vi "诊断标定3.vi"(8 "CAN端口":u16(ring), 9 "设备索引号":u16(ring), 10 "CAN卡类型":u32(ring)=21) -> ()   [LabVIEW 2013] (continued)
            n2342 = global write "EV05全局变量1.vi" "流控帧 2"(TRUE ("流控帧 2")) -> ()
            n2343 = local write "写?"(FALSE ("写?")) -> ()
            n2344 = local write "消除"(TRUE ("消除")) -> ()
          }
          frame #2 {
            n2345 = flat-sequence {
              tunnel: [w2891] -> w2890
              tunnel: w2890 -> [w2898]
              frame #0 {
                n2346 = while {
                  tunnel: [w2892] -> w2891
                  i -> [w2896]
                  stop <- w2893 stop-if-true
                  n2347 = local read "继电器超时处理"() -> (w2892:bool)
                  n2348 = Greater Or Equal?(x=w2896, y=20) -> (x >= y?=w2894:bool)
                  n2349 = Wait Until Next ms Multiple(millisecond multiple=u32 100 ("毫秒倍数")) -> ()  [unwired: 1 out]
                  n2350 = Or(x=w2892, y=w2894) -> (x .or. y?=w2893:bool)
                }
              }
              frame #1 {
                n2351 = case shown="假" w2898 {
                  frame False {
                    n2352 = local read "负级继电器"() -> (w2899:bool)
                    n2353 = Not(x=w2899) -> (.not. x?=w2900:bool)
                    n2354 = local write "负级继电器"(w2900) -> ()
                    n2355 = One Button Dialog(message="继电器处理超时" ("消息"), button name ("OK")="是" ("按钮名称（“确定”）")) -> ()  [unwired: 1 out]
                  }
                  frame True {
                  }
                }
              }
            }
          }
        }
      }
      event "预充电继电器": Value Change {
        n2356 = event-data() -> ("NewVal"=w2903:bool)  [unwired: 6 out]
        n2357 = stacked-sequence {
          tunnel: w2903 -> [_ w2916 _]
          frame #0 {
            w2907 = FALSE ("继电器超时处理")
            n2358 = local write "继电器超时处理"(w2907) -> ()
            n2359 = local write "正级继电器 3"(w2907) -> ()
            n2360 = global write "EV05全局变量1.vi" "流控帧"(FALSE ("流控帧")) -> ()
            n2361 = local write "主从选择"(enum32{"主板", "从板"}."主板" ("主从选择")) -> ()
          }
          frame #1 {
            n2362 = case shown="假" w2916 {
              selector: w2916 -> [w2930 w2950]
              tunnel: [w2929 w2949] -> w2915
              tunnel: [w2918 w2938] -> w2910
              frame False {
                w2926 = 256.0 ("y")
                w2918 = u32 1 ("命令序号")
                w2929 = u8 192 ("命令")
                n2363 = local read "动作保持时间"() -> (w2927:dbl)
                n2364 = Quotient & Remainder(x=w2927, y=w2926) -> (x-y*floor(x/y)=w2919:dbl, floor(x/y)=w2923:dbl)
                n2365 = Quotient & Remainder(x=w2923, y=w2926) -> (x-y*floor(x/y)=w2920:dbl, floor(x/y)=w2924:dbl)
                n2366 = Quotient & Remainder(x=w2924, y=w2926) -> (x-y*floor(x/y)=w2921:dbl, floor(x/y)=w2925:dbl)
                n2367 = Quotient & Remainder(x=w2925, y=w2926) -> (x-y*floor(x/y)=w2922:dbl)  [unwired: 1 out]
                n2368 = Boolean To (0,1)(Boolean=w2930) -> (0, 1=w2928:i16)
                n2369 = local read "设备索引号"() -> (w2935:u16)
                n2370 = local read "CAN卡类型"() -> (w2936:u32)
                n2371 = local read "CAN端口"() -> (w2934:u16)
                n2372 = Build Array(i16 3 ("元素"), w2928, w2922, w2921, w2920, w2919, 0.0 ("元素")) -> (w2932:dbl[])
                n2373 = call "多帧发送机制(EV05).vi"("can卡类型"=w2936, "设备索引号"=w2935, "CAN端口"=w2934, "命令"=w2929, "板号"=u8 0, "命令序号"=w2918, "输入数据"=w2932) -> ()  [unwired: 1 in, 12 out]
              }
              frame True {
                w2946 = 256.0 ("y")
                w2938 = u32 1 ("命令序号")
                w2949 = u8 192 ("命令")
                n2374 = local read "动作保持时间"() -> (w2947:dbl)
                n2375 = Quotient & Remainder(x=w2947, y=w2946) -> (x-y*floor(x/y)=w2939:dbl, floor(x/y)=w2943:dbl)
                n2376 = Quotient & Remainder(x=w2943, y=w2946) -> (x-y*floor(x/y)=w2940:dbl, floor(x/y)=w2944:dbl)
                n2377 = Quotient & Remainder(x=w2944, y=w2946) -> (x-y*floor(x/y)=w2941:dbl, floor(x/y)=w2945:dbl)
                n2378 = Quotient & Remainder(x=w2945, y=w2946) -> (x-y*floor(x/y)=w2942:dbl)  [unwired: 1 out]
                n2379 = Boolean To (0,1)(Boolean=w2950) -> (0, 1=w2948:i16)
                n2380 = local read "设备索引号"() -> (w2955:u16)
                n2381 = local read "CAN卡类型"() -> (w2956:u32)
                n2382 = local read "CAN端口"() -> (w2954:u16)
                n2383 = Build Array(i16 3 ("元素"), w2948, w2942, w2941, w2940, w2939, 0.0 ("元素")) -> (w2952:dbl[])
                n2384 = call "多帧发送机制(EV05).vi"("can卡类型"=w2956, "设备索引号"=w2955, "CAN端口"=w2954, "命令"=w2949, "板号"=u8 0, "命令序号"=w2938, "输入数据"=w2952) -> ()  [unwired: 1 in, 12 out]
              }
            }
            n2385 = local write "命令序号"(w2910) -> ()
            n2386 = local write "清BUFF"(FALSE ("清BUFF")) -> ()
            n2387 = local write "控制1"(TRUE ("控制1")) -> ()
            n2388 = global write "EV05全局变量1.vi" "流控帧 2"(TRUE ("流控帧 2")) -> ()
            n2389 = local write "消除"(TRUE ("消除")) -> ()
            n2390 = local write "命令"(w2915) -> ()
            n2391 = local write "写?"(FALSE ("写?")) -> ()
          }
          frame #2 {
            n2392 = flat-sequence {
              tunnel: [w2958] -> w2957
              tunnel: w2957 -> [w2965]
              frame #0 {
                n2393 = while {
                  tunnel: [w2959] -> w2958
                  i -> [w2963]
                  stop <- w2960 stop-if-true
                  n2394 = local read "继电器超时处理"() -> (w2959:bool)
                  n2395 = Greater Or Equal?(x=w2963, y=20) -> (x >= y?=w2961:bool)
                  n2396 = Wait Until Next ms Multiple(millisecond multiple=u32 100 ("毫秒倍数")) -> ()  [unwired: 1 out]
                  n2397 = Or(x=w2959, y=w2961) -> (x .or. y?=w2960:bool)
                }
              }
              frame #1 {
                n2398 = case shown="假" w2965 {
                  frame False {
                    n2399 = local read "预充电继电器"() -> (w2966:bool)
                    n2400 = Not(x=w2966) -> (.not. x?=w2967:bool)
                    n2401 = local write "预充电继电器"(w2967) -> ()
                    n2402 = One Button Dialog(message="继电器处理超时" ("消息"), button name ("OK")="是" ("按钮名称（“确定”）")) -> ()  [unwired: 1 out]
                  }
                  frame True {
                  }
                }
              }
            }
          }
        }
      }
      event "加热继电器": Value Change {
        n2403 = event-data() -> ("NewVal"=w2970:bool)  [unwired: 6 out]
        n2404 = stacked-sequence {
          tunnel: w2970 -> [_ w2983 _]
          frame #0 {
            w2974 = FALSE ("继电器超时处理")
            n2405 = local write "继电器超时处理"(w2974) -> ()
            n2406 = local write "正级继电器 5"(w2974) -> ()
            n2407 = global write "EV05全局变量1.vi" "流控帧"(FALSE ("流控帧")) -> ()
            n2408 = local write "主从选择"(enum32{"主板", "从板"}."主板" ("主从选择")) -> ()
          }
          frame #1 {
            n2409 = case shown="假" w2983 {
              selector: w2983 -> [w2997 w3017]
              tunnel: [w2996 w3016] -> w2982
              tunnel: [w2985 w3005] -> w2977
              frame False {
                w2993 = 256.0 ("y")
                w2985 = u32 1 ("命令序号")
                w2996 = u8 192 ("命令")
                n2410 = local read "动作保持时间"() -> (w2994:dbl)
                n2411 = Quotient & Remainder(x=w2994, y=w2993) -> (x-y*floor(x/y)=w2986:dbl, floor(x/y)=w2990:dbl)
                n2412 = Quotient & Remainder(x=w2990, y=w2993) -> (x-y*floor(x/y)=w2987:dbl, floor(x/y)=w2991:dbl)
                n2413 = Quotient & Remainder(x=w2991, y=w2993) -> (x-y*floor(x/y)=w2988:dbl, floor(x/y)=w2992:dbl)
                n2414 = Quotient & Remainder(x=w2992, y=w2993) -> (x-y*floor(x/y)=w2989:dbl)  [unwired: 1 out]
                n2415 = Boolean To (0,1)(Boolean=w2997) -> (0, 1=w2995:i16)
                n2416 = local read "设备索引号"() -> (w3002:u16)
                n2417 = local read "CAN卡类型"() -> (w3003:u32)
                n2418 = local read "CAN端口"() -> (w3001:u16)
                n2419 = Build Array(i16 4 ("元素"), w2995, w2989, w2988, w2987, w2986, 0.0 ("元素")) -> (w2999:dbl[])
                n2420 = call "多帧发送机制(EV05).vi"("can卡类型"=w3003, "设备索引号"=w3002, "CAN端口"=w3001, "命令"=w2996, "板号"=u8 0, "命令序号"=w2985, "输入数据"=w2999) -> ()  [unwired: 1 in, 12 out]
              }
              frame True {
                w3013 = 256.0 ("y")
                w3005 = u32 1 ("命令序号")
                w3016 = u8 192 ("命令")
                n2421 = local read "动作保持时间"() -> (w3014:dbl)
                n2422 = Quotient & Remainder(x=w3014, y=w3013) -> (x-y*floor(x/y)=w3006:dbl, floor(x/y)=w3010:dbl)
                n2423 = Quotient & Remainder(x=w3010, y=w3013) -> (x-y*floor(x/y)=w3007:dbl, floor(x/y)=w3011:dbl)
                n2424 = Quotient & Remainder(x=w3011, y=w3013) -> (x-y*floor(x/y)=w3008:dbl, floor(x/y)=w3012:dbl)
                n2425 = Quotient & Remainder(x=w3012, y=w3013) -> (x-y*floor(x/y)=w3009:dbl)  [unwired: 1 out]
                n2426 = Boolean To (0,1)(Boolean=w3017) -> (0, 1=w3015:i16)
                n2427 = local read "设备索引号"() -> (w3022:u16)
                n2428 = local read "CAN卡类型"() -> (w3023:u32)
                n2429 = local read "CAN端口"() -> (w3021:u16)
                n2430 = Build Array(i16 4 ("元素"), w3015, w3009, w3008, w3007, w3006, 0.0 ("元素")) -> (w3019:dbl[])
                n2431 = call "多帧发送机制(EV05).vi"("can卡类型"=w3023, "设备索引号"=w3022, "CAN端口"=w3021, "命令"=w3016, "板号"=u8 0, "命令序号"=w3005, "输入数据"=w3019) -> ()  [unwired: 1 in, 12 out]
              }
            }
            n2432 = local write "命令序号"(w2977) -> ()
            n2433 = local write "清BUFF"(FALSE ("清BUFF")) -> ()
            n2434 = local write "命令"(w2982) -> ()
            n2435 = local write "控制1"(TRUE ("控制1")) -> ()
            n2436 = local write "写?"(FALSE ("写?")) -> ()
            n2437 = global write "EV05全局变量1.vi" "流控帧 2"(TRUE ("流控帧 2")) -> ()
            n2438 = local write "消除"(TRUE ("消除")) -> ()
          }
          frame #2 {
            n2439 = flat-sequence {
              tunnel: [w3025] -> w3024
              tunnel: w3024 -> [w3032]
              frame #0 {
                n2440 = while {
                  tunnel: [w3026] -> w3025
                  i -> [w3030]
                  stop <- w3027 stop-if-true
                  n2441 = local read "继电器超时处理"() -> (w3026:bool)
                  n2442 = Greater Or Equal?(x=w3030, y=20) -> (x >= y?=w3028:bool)
                  n2443 = Wait Until Next ms Multiple(millisecond multiple=u32 100 ("毫秒倍数")) -> ()  [unwired: 1 out]
                  n2444 = Or(x=w3026, y=w3028) -> (x .or. y?=w3027:bool)
                }
              }
              frame #1 {
                n2445 = case shown="假" w3032 {
                  frame False {
                    n2446 = local read "加热继电器"() -> (w3033:bool)
                    n2447 = Not(x=w3033) -> (.not. x?=w3034:bool)
                    n2448 = local write "加热继电器"(w3034) -> ()
                    n2449 = One Button Dialog(message="继电器处理超时" ("消息"), button name ("OK")="是" ("按钮名称（“确定”）")) -> ()  [unwired: 1 out]
                  }
                  frame True {
                  }
                }
              }
            }
          }
        }
      }
      event "充电继电器": Value Change {
        n2450 = event-data() -> ("NewVal"=w3037:bool)  [unwired: 6 out]
        n2451 = stacked-sequence {
          tunnel: w3037 -> [_ w3050 _]
          frame #0 {
            w3041 = FALSE ("继电器超时处理")
            n2452 = local write "主从选择"(enum32{"主板", "从板"}."主板" ("主从选择")) -> ()
            n2453 = global write "EV05全局变量1.vi" "流控帧"(FALSE ("流控帧")) -> ()
            n2454 = local write "继电器超时处理"(w3041) -> ()
            n2455 = local write "正级继电器 4"(w3041) -> ()
          }
          frame #1 {
            n2456 = case shown="假" w3050 {
              selector: w3050 -> [w3064 w3084]
              tunnel: [w3063 w3083] -> w3049
              tunnel: [w3052 w3072] -> w3044
              frame False {
                w3060 = 256.0 ("y")
                w3052 = u32 1 ("命令序号")
                w3063 = u8 192 ("命令")
                n2457 = local read "动作保持时间"() -> (w3061:dbl)
                n2458 = Quotient & Remainder(x=w3061, y=w3060) -> (x-y*floor(x/y)=w3053:dbl, floor(x/y)=w3057:dbl)
                n2459 = Quotient & Remainder(x=w3057, y=w3060) -> (x-y*floor(x/y)=w3054:dbl, floor(x/y)=w3058:dbl)
                n2460 = Quotient & Remainder(x=w3058, y=w3060) -> (x-y*floor(x/y)=w3055:dbl, floor(x/y)=w3059:dbl)
                n2461 = Quotient & Remainder(x=w3059, y=w3060) -> (x-y*floor(x/y)=w3056:dbl)  [unwired: 1 out]
                n2462 = Boolean To (0,1)(Boolean=w3064) -> (0, 1=w3062:i16)
                n2463 = local read "设备索引号"() -> (w3069:u16)
                n2464 = local read "CAN卡类型"() -> (w3070:u32)
                n2465 = local read "CAN端口"() -> (w3068:u16)
                n2466 = Build Array(i16 5 ("元素"), w3062, w3056, w3055, w3054, w3053, 0.0 ("元素")) -> (w3066:dbl[])
                n2467 = call "多帧发送机制(EV05).vi"("can卡类型"=w3070, "设备索引号"=w3069, "CAN端口"=w3068, "命令"=w3063, "板号"=u8 0, "命令序号"=w3052, "输入数据"=w3066) -> ()  [unwired: 1 in, 12 out]
              }
              frame True {
                w3080 = 256.0 ("y")
                w3072 = u32 1 ("命令序号")
                w3083 = u8 192 ("命令")
                n2468 = local read "动作保持时间"() -> (w3081:dbl)
                n2469 = Quotient & Remainder(x=w3081, y=w3080) -> (x-y*floor(x/y)=w3073:dbl, floor(x/y)=w3077:dbl)
                n2470 = Quotient & Remainder(x=w3077, y=w3080) -> (x-y*floor(x/y)=w3074:dbl, floor(x/y)=w3078:dbl)
                n2471 = Quotient & Remainder(x=w3078, y=w3080) -> (x-y*floor(x/y)=w3075:dbl, floor(x/y)=w3079:dbl)
                n2472 = Quotient & Remainder(x=w3079, y=w3080) -> (x-y*floor(x/y)=w3076:dbl)  [unwired: 1 out]
                n2473 = Boolean To (0,1)(Boolean=w3084) -> (0, 1=w3082:i16)
                n2474 = local read "设备索引号"() -> (w3089:u16)
                n2475 = local read "CAN卡类型"() -> (w3090:u32)
                n2476 = local read "CAN端口"() -> (w3088:u16)
                n2477 = Build Array(i16 5 ("元素"), w3082, w3076, w3075, w3074, w3073, 0.0 ("元素")) -> (w3086:dbl[])
                n2478 = call "多帧发送机制(EV05).vi"("can卡类型"=w3090, "设备索引号"=w3089, "CAN端口"=w3088, "命令"=w3083, "板号"=u8 0, "命令序号"=w3072, "输入数据"=w3086) -> ()  [unwired: 1 in, 12 out]
              }
            }
            n2479 = local write "命令序号"(w3044) -> ()
            n2480 = local write "命令"(w3049) -> ()
            n2481 = local write "清BUFF"(FALSE ("清BUFF")) -> ()
            n2482 = local write "控制1"(TRUE ("控制1")) -> ()
            n2483 = global write "EV05全局变量1.vi" "流控帧 2"(TRUE ("流控帧 2")) -> ()
            n2484 = local write "写?"(FALSE ("写?")) -> ()
            n2485 = local write "消除"(TRUE ("消除")) -> ()
          }
          frame #2 {
            n2486 = flat-sequence {
              tunnel: [w3092] -> w3091
              tunnel: w3091 -> [w3099]
              frame #0 {
                n2487 = while {
                  tunnel: [w3093] -> w3092
                  i -> [w3097]
                  stop <- w3094 stop-if-true
                  n2488 = local read "继电器超时处理"() -> (w3093:bool)
                  n2489 = Greater Or Equal?(x=w3097, y=20) -> (x >= y?=w3095:bool)
                  n2490 = Wait Until Next ms Multiple(millisecond multiple=u32 100 ("毫秒倍数")) -> ()  [unwired: 1 out]
                  n2491 = Or(x=w3093, y=w3095) -> (x .or. y?=w3094:bool)
                }
              }
              frame #1 {
                n2492 = case shown="假" w3099 {
                  frame False {
                    n2493 = local read "充电继电器"() -> (w3100:bool)
                    n2494 = Not(x=w3100) -> (.not. x?=w3101:bool)
                    n2495 = local write "充电继电器"(w3101) -> ()
                    n2496 = One Button Dialog(message="继电器处理超时" ("消息"), button name ("OK")="是" ("按钮名称（“确定”）")) -> ()  [unwired: 1 out]
                  }
                  frame True {
                  }
                }
              }
            }
          }
        }
      }
      event "风机继电器": Value Change {
        n2497 = event-data() -> ("NewVal"=w3104:bool)  [unwired: 6 out]
        n2498 = stacked-sequence {
          tunnel: w3104 -> [_ w3117 _]
          frame #0 {
            w3108 = FALSE ("继电器超时处理")
            n2499 = local write "继电器超时处理"(w3108) -> ()
            n2500 = local write "正级继电器 6"(w3108) -> ()
            n2501 = global write "EV05全局变量1.vi" "流控帧"(FALSE ("流控帧")) -> ()
            n2502 = local write "主从选择"(enum32{"主板", "从板"}."主板" ("主从选择")) -> ()
          }
          frame #1 {
            n2503 = case shown="真" w3117 {
              selector: w3117 -> [w3131 w3151]
              tunnel: [w3130 w3150] -> w3116
              tunnel: [w3119 w3139] -> w3111
              frame True {
                w3127 = 256.0 ("y")
                w3119 = u32 1 ("命令序号")
                w3130 = u8 192 ("命令")
                n2504 = local read "动作保持时间"() -> (w3128:dbl)
                n2505 = Quotient & Remainder(x=w3128, y=w3127) -> (x-y*floor(x/y)=w3120:dbl, floor(x/y)=w3124:dbl)
                n2506 = Quotient & Remainder(x=w3124, y=w3127) -> (x-y*floor(x/y)=w3121:dbl, floor(x/y)=w3125:dbl)
                n2507 = Quotient & Remainder(x=w3125, y=w3127) -> (x-y*floor(x/y)=w3122:dbl, floor(x/y)=w3126:dbl)
                n2508 = Boolean To (0,1)(Boolean=w3131) -> (0, 1=w3129:i16)
                n2509 = local read "设备索引号"() -> (w3136:u16)
                n2510 = local read "CAN卡类型"() -> (w3137:u32)
                n2511 = Quotient & Remainder(x=w3126, y=w3127) -> (x-y*floor(x/y)=w3123:dbl)  [unwired: 1 out]
                n2512 = local read "CAN端口"() -> (w3135:u16)
                n2513 = Build Array(i16 6 ("元素"), w3129, w3123, w3122, w3121, w3120, 0.0 ("元素")) -> (w3133:dbl[])
                n2514 = call "多帧发送机制(EV05).vi"("can卡类型"=w3137, "设备索引号"=w3136, "CAN端口"=w3135, "命令"=w3130, "板号"=u8 0, "命令序号"=w3119, "输入数据"=w3133) -> ()  [unwired: 1 in, 12 out]
              }
              frame False {
                w3147 = 256.0 ("y")
                w3139 = u32 1 ("命令序号")
                w3150 = u8 192 ("命令")
                n2515 = local read "动作保持时间"() -> (w3148:dbl)
                n2516 = Quotient & Remainder(x=w3148, y=w3147) -> (x-y*floor(x/y)=w3140:dbl, floor(x/y)=w3144:dbl)
                n2517 = Quotient & Remainder(x=w3144, y=w3147) -> (x-y*floor(x/y)=w3141:dbl, floor(x/y)=w3145:dbl)
                n2518 = Quotient & Remainder(x=w3145, y=w3147) -> (x-y*floor(x/y)=w3142:dbl, floor(x/y)=w3146:dbl)
                n2519 = Boolean To (0,1)(Boolean=w3151) -> (0, 1=w3149:i16)
                n2520 = local read "设备索引号"() -> (w3156:u16)
                n2521 = local read "CAN卡类型"() -> (w3157:u32)
                n2522 = Quotient & Remainder(x=w3146, y=w3147) -> (x-y*floor(x/y)=w3143:dbl)  [unwired: 1 out]
                n2523 = local read "CAN端口"() -> (w3155:u16)
                n2524 = Build Array(i16 6 ("元素"), w3149, w3143, w3142, w3141, w3140, 0.0 ("元素")) -> (w3153:dbl[])
                n2525 = call "多帧发送机制(EV05).vi"("can卡类型"=w3157, "设备索引号"=w3156, "CAN端口"=w3155, "命令"=w3150, "板号"=u8 0, "命令序号"=w3139, "输入数据"=w3153) -> ()  [unwired: 1 in, 12 out]
              }
            }
            n2526 = local write "命令序号"(w3111) -> ()
            n2527 = local write "命令"(w3116) -> ()
            n2528 = local write "清BUFF"(FALSE ("清BUFF")) -> ()
            n2529 = local write "控制1"(TRUE ("控制1")) -> ()
            n2530 = global write "EV05全局变量1.vi" "流控帧 2"(TRUE ("流控帧 2")) -> ()
            n2531 = local write "写?"(FALSE ("写?")) -> ()
            n2532 = local write "消除"(TRUE ("消除")) -> ()
          }
          frame #2 {
            n2533 = flat-sequence {
              tunnel: [w3159] -> w3158
              tunnel: w3158 -> [w3166]
              frame #0 {
                n2534 = while {
                  tunnel: [w3160] -> w3159
                  i -> [w3164]
                  stop <- w3161 stop-if-true
                  n2535 = local read "继电器超时处理"() -> (w3160:bool)
                  n2536 = Greater Or Equal?(x=w3164, y=20) -> (x >= y?=w3162:bool)
                  n2537 = Wait Until Next ms Multiple(millisecond multiple=u32 100 ("毫秒倍数")) -> ()  [unwired: 1 out]
                  n2538 = Or(x=w3160, y=w3162) -> (x .or. y?=w3161:bool)
                }
              }
              frame #1 {
                n2539 = case shown="假" w3166 {
                  frame False {
                    n2540 = local read "风机继电器"() -> (w3167:bool)
                    n2541 = Not(x=w3167) -> (.not. x?=w3168:bool)
                    n2542 = local write "风机继电器"(w3168) -> ()
                    n2543 = One Button Dialog(message="继电器处理超时" ("消息"), button name ("OK")="是" ("按钮名称（“确定”）")) -> ()  [unwired: 1 out]
                  }
                  frame True {
                  }
                }
              }
            }
          }
        }
      }
      event "加热继电器(从)": Value Change {
        n2544 = event-data() -> ("NewVal"=w3171:bool)  [unwired: 6 out]
        n2545 = stacked-sequence {
          tunnel: w3171 -> [_ w3185 _]
          frame #0 {
            w3175 = FALSE ("继电器超时处理")
            n2546 = local write "正级继电器 7"(w3175) -> ()
            n2547 = local write "继电器超时处理"(w3175) -> ()
            n2548 = global write "EV05全局变量1.vi" "流控帧"(FALSE ("流控帧")) -> ()
            n2549 = local write "主从选择"(enum32{"主板", "从板"}."从板" ("主从选择")) -> ()
          }
          frame #1 {
            n2550 = case shown="真" w3185 {
              selector: w3185 -> [w3200 w3220]
              tunnel: [w3199 w3219] -> w3184
              tunnel: [w3198 w3218] -> w3178
              tunnel: [w3187 w3207] -> w3179
              frame True {
                w3195 = 256.0 ("y")
                w3187 = u32 1 ("命令序号")
                w3199 = u8 192 ("命令")
                n2551 = local read "动作保持时间"() -> (w3196:dbl)
                n2552 = Quotient & Remainder(x=w3196, y=w3195) -> (x-y*floor(x/y)=w3188:dbl, floor(x/y)=w3192:dbl)
                n2553 = Quotient & Remainder(x=w3192, y=w3195) -> (x-y*floor(x/y)=w3189:dbl, floor(x/y)=w3193:dbl)
                n2554 = Quotient & Remainder(x=w3193, y=w3195) -> (x-y*floor(x/y)=w3190:dbl, floor(x/y)=w3194:dbl)
                n2555 = Quotient & Remainder(x=w3194, y=w3195) -> (x-y*floor(x/y)=w3191:dbl)  [unwired: 1 out]
                n2556 = Boolean To (0,1)(Boolean=w3200) -> (0, 1=w3197:i16)
                n2557 = local read "设备索引号"() -> (w3204:u16)
                n2558 = local read "CAN卡类型"() -> (w3205:u32)
                n2559 = local read "从板板号"() -> (w3198:u8)
                n2560 = local read "CAN端口"() -> (w3203:u16)
                n2561 = Build Array(i16 7 ("元素"), w3197, w3191, w3190, w3189, w3188, 0.0 ("元素")) -> (w3202:dbl[])
                n2562 = call "多帧发送机制(EV05).vi"("can卡类型"=w3205, "设备索引号"=w3204, "CAN端口"=w3203, "命令"=w3199, "板号"=w3198, "命令序号"=w3187, "输入数据"=w3202) -> ()  [unwired: 1 in, 12 out]
              }
              frame False {
                w3215 = 256.0 ("y")
                w3207 = u32 1 ("命令序号")
                w3219 = u8 192 ("命令")
                n2563 = local read "动作保持时间"() -> (w3216:dbl)
                n2564 = Quotient & Remainder(x=w3216, y=w3215) -> (x-y*floor(x/y)=w3208:dbl, floor(x/y)=w3212:dbl)
                n2565 = Quotient & Remainder(x=w3212, y=w3215) -> (x-y*floor(x/y)=w3209:dbl, floor(x/y)=w3213:dbl)
                n2566 = Quotient & Remainder(x=w3213, y=w3215) -> (x-y*floor(x/y)=w3210:dbl, floor(x/y)=w3214:dbl)
                n2567 = Quotient & Remainder(x=w3214, y=w3215) -> (x-y*floor(x/y)=w3211:dbl)  [unwired: 1 out]
                n2568 = Boolean To (0,1)(Boolean=w3220) -> (0, 1=w3217:i16)
                n2569 = local read "设备索引号"() -> (w3224:u16)
                n2570 = local read "CAN卡类型"() -> (w3225:u32)
                n2571 = local read "从板板号"() -> (w3218:u8)
                n2572 = local read "CAN端口"() -> (w3223:u16)
                n2573 = Build Array(i16 7 ("元素"), w3217, w3211, w3210, w3209, w3208, 0.0 ("元素")) -> (w3222:dbl[])
                n2574 = call "多帧发送机制(EV05).vi"("can卡类型"=w3225, "设备索引号"=w3224, "CAN端口"=w3223, "命令"=w3219, "板号"=w3218, "命令序号"=w3207, "输入数据"=w3222) -> ()  [unwired: 1 in, 12 out]
              }
            }
            n2575 = local write "从板板号"(w3178) -> ()
            n2576 = local write "命令序号"(w3179) -> ()
            n2577 = local write "命令"(w3184) -> ()
            n2578 = local write "清BUFF"(FALSE ("清BUFF")) -> ()
            n2579 = local write "写?"(FALSE ("写?")) -> ()
            n2580 = local write "控制1"(TRUE ("控制1")) -> ()
            n2581 = global write "EV05全局变量1.vi" "流控帧 2"(TRUE ("流控帧 2")) -> ()
            n2582 = local write "消除"(TRUE ("消除")) -> ()
          }
          frame #2 {
            n2583 = flat-sequence {
              tunnel: [w3227] -> w3226
              tunnel: w3226 -> [w3234]
              frame #0 {
                n2584 = while {
                  tunnel: [w3228] -> w3227
                  i -> [w3232]
                  stop <- w3229 stop-if-true
                  n2585 = local read "继电器超时处理"() -> (w3228:bool)
                  n2586 = Greater Or Equal?(x=w3232, y=20) -> (x >= y?=w3230:bool)
                  n2587 = Wait Until Next ms Multiple(millisecond multiple=u32 100 ("毫秒倍数")) -> ()  [unwired: 1 out]
                  n2588 = Or(x=w3228, y=w3230) -> (x .or. y?=w3229:bool)
                }
              }
              frame #1 {
                n2589 = case shown="假" w3234 {
                  frame False {
                    n2590 = local read "加热继电器(从)"() -> (w3236:bool)
                    n2591 = Not(x=w3236) -> (.not. x?=w3235:bool)
                    n2592 = local write "加热继电器(从)"(w3235) -> ()
                    n2593 = One Button Dialog(message="继电器处理超时" ("消息"), button name ("OK")="是" ("按钮名称（“确定”）")) -> ()  [unwired: 1 out]
                  }
                  frame True {
                  }
                }
              }
            }
          }
        }
      }
      event "风机继电器(从)": Value Change {
        n2594 = event-data() -> ("NewVal"=w3239:bool)  [unwired: 6 out]
        n2595 = stacked-sequence {
          tunnel: w3239 -> [_ w3253 _]
          frame #0 {
            w3243 = FALSE ("继电器超时处理")
            n2596 = local write "继电器超时处理"(w3243) -> ()
            n2597 = local write "正级继电器 8"(w3243) -> ()
            n2598 = global write "EV05全局变量1.vi" "流控帧"(FALSE ("流控帧")) -> ()
            n2599 = local write "主从选择"(enum32{"主板", "从板"}."从板" ("主从选择")) -> ()
          }
          frame #1 {
            n2600 = case shown="假" w3253 {
              selector: w3253 -> [w3268 w3288]
              tunnel: [w3267 w3287] -> w3252
              tunnel: [w3266 w3286] -> w3246
              tunnel: [w3255 w3275] -> w3247
              frame False {
                w3263 = 256.0 ("y")
                w3255 = u32 1 ("命令序号")
                w3267 = u8 192 ("命令")
                n2601 = local read "动作保持时间"() -> (w3264:dbl)
                n2602 = Quotient & Remainder(x=w3264, y=w3263) -> (x-y*floor(x/y)=w3256:dbl, floor(x/y)=w3260:dbl)
                n2603 = Quotient & Remainder(x=w3260, y=w3263) -> (x-y*floor(x/y)=w3257:dbl, floor(x/y)=w3261:dbl)
                n2604 = Quotient & Remainder(x=w3261, y=w3263) -> (x-y*floor(x/y)=w3258:dbl, floor(x/y)=w3262:dbl)
                n2605 = Quotient & Remainder(x=w3262, y=w3263) -> (x-y*floor(x/y)=w3259:dbl)  [unwired: 1 out]
                n2606 = local read "设备索引号"() -> (w3272:u16)
                n2607 = local read "CAN卡类型"() -> (w3273:u32)
                n2608 = local read "从板板号"() -> (w3266:u8)
                n2609 = Boolean To (0,1)(Boolean=w3268) -> (0, 1=w3265:i16)
                n2610 = local read "CAN端口"() -> (w3271:u16)
                n2611 = Build Array(i16 8 ("元素"), w3265, w3259, w3258, w3257, w3256, 0.0 ("元素")) -> (w3270:dbl[])
                n2612 = call "多帧发送机制(EV05).vi"("can卡类型"=w3273, "设备索引号"=w3272, "CAN端口"=w3271, "命令"=w3267, "板号"=w3266, "命令序号"=w3255, "输入数据"=w3270) -> ()  [unwired: 1 in, 12 out]
              }
              frame True {
                w3283 = 256.0 ("y")
                w3275 = u32 1 ("命令序号")
                w3287 = u8 192 ("命令")
                n2613 = local read "动作保持时间"() -> (w3284:dbl)
                n2614 = Quotient & Remainder(x=w3284, y=w3283) -> (x-y*floor(x/y)=w3276:dbl, floor(x/y)=w3280:dbl)
                n2615 = Quotient & Remainder(x=w3280, y=w3283) -> (x-y*floor(x/y)=w3277:dbl, floor(x/y)=w3281:dbl)
                n2616 = Quotient & Remainder(x=w3281, y=w3283) -> (x-y*floor(x/y)=w3278:dbl, floor(x/y)=w3282:dbl)
                n2617 = Quotient & Remainder(x=w3282, y=w3283) -> (x-y*floor(x/y)=w3279:dbl)  [unwired: 1 out]
                n2618 = local read "设备索引号"() -> (w3292:u16)
                n2619 = local read "CAN卡类型"() -> (w3293:u32)
                n2620 = local read "从板板号"() -> (w3286:u8)
                n2621 = Boolean To (0,1)(Boolean=w3288) -> (0, 1=w3285:i16)
                n2622 = local read "CAN端口"() -> (w3291:u16)
                n2623 = Build Array(i16 8 ("元素"), w3285, w3279, w3278, w3277, w3276, 0.0 ("元素")) -> (w3290:dbl[])
                n2624 = call "多帧发送机制(EV05).vi"("can卡类型"=w3293, "设备索引号"=w3292, "CAN端口"=w3291, "命令"=w3287, "板号"=w3286, "命令序号"=w3275, "输入数据"=w3290) -> ()  [unwired: 1 in, 12 out]
              }
            }
            n2625 = local write "从板板号"(w3246) -> ()
            n2626 = local write "清BUFF"(FALSE ("清BUFF")) -> ()
            n2627 = local write "命令序号"(w3247) -> ()
            n2628 = local write "命令"(w3252) -> ()
            n2629 = local write "控制1"(TRUE ("控制1")) -> ()
            n2630 = local write "写?"(FALSE ("写?")) -> ()
            n2631 = local write "消除"(TRUE ("消除")) -> ()
            n2632 = global write "EV05全局变量1.vi" "流控帧 2"(TRUE ("流控帧 2")) -> ()
          }
          frame #2 {
            n2633 = flat-sequence {
              tunnel: [w3295] -> w3294
              tunnel: w3294 -> [w3302]
              frame #0 {
                n2634 = while {
                  tunnel: [w3296] -> w3295
                  i -> [w3300]
                  stop <- w3297 stop-if-true
                  n2635 = local read "继电器超时处理"() -> (w3296:bool)
                  n2636 = Greater Or Equal?(x=w3300, y=20) -> (x >= y?=w3298:bool)
                  n2637 = Wait Until Next ms Multiple(millisecond multiple=u32 100 ("毫秒倍数")) -> ()  [unwired: 1 out]
                  n2638 = Or(x=w3296, y=w3298) -> (x .or. y?=w3297:bool)
                }
              }
              frame #1 {
                n2639 = case shown="假" w3302 {
                  frame False {
                    n2640 = local read "风机继电器(从)"() -> (w3304:bool)
                    n2641 = Not(x=w3304) -> (.not. x?=w3303:bool)
                    n2642 = local write "风机继电器(从)"(w3303) -> ()
                    n2643 = One Button Dialog(message="继电器处理超时" ("消息"), button name ("OK")="是" ("按钮名称（“确定”）")) -> ()  [unwired: 1 out]
                  }
                  frame True {
                  }
                }
              }
            }
          }
        }
      }
      event "DO1": Value Change {
        n2644 = event-data() -> ("NewVal"=w3307:bool)  [unwired: 6 out]
        n2645 = stacked-sequence {
          tunnel: w3307 -> [_ w3320 _]
          frame #0 {
            w3310 = FALSE ("清BUFF")
            n2646 = local write "继电器超时处理"(FALSE ("继电器超时处理")) -> ()
            n2647 = local write "清BUFF"(w3310) -> ()
            n2648 = local write "正级继电器 9"(w3310) -> ()
            n2649 = local write "主从选择"(enum32{"主板", "从板"}."主板" ("主从选择")) -> ()
          }
          frame #1 {
            n2650 = case shown="真" w3320 {
              selector: w3320 -> [w3335 w3355]
              tunnel: [w3334 w3354] -> w3319
              tunnel: [w3322 w3342] -> w3314
              frame False {
                w3330 = 256.0 ("y")
                w3322 = u32 2 ("命令序号")
                w3334 = u8 192 ("命令")
                n2651 = local read "动作保持时间"() -> (w3331:dbl)
                n2652 = Quotient & Remainder(x=w3331, y=w3330) -> (x-y*floor(x/y)=w3323:dbl, floor(x/y)=w3327:dbl)
                n2653 = Quotient & Remainder(x=w3327, y=w3330) -> (x-y*floor(x/y)=w3324:dbl, floor(x/y)=w3328:dbl)
                n2654 = Quotient & Remainder(x=w3328, y=w3330) -> (x-y*floor(x/y)=w3325:dbl, floor(x/y)=w3329:dbl)
                n2655 = local read "设备索引号"() -> (w3339:u16)
                n2656 = local read "CAN卡类型"() -> (w3340:u32)
                n2657 = local read "CAN端口"() -> (w3338:u16)
                n2658 = Boolean To (0,1)(Boolean=w3335) -> (0, 1=w3332:i16)
                n2659 = Quotient & Remainder(x=w3329, y=w3330) -> (x-y*floor(x/y)=w3326:dbl)  [unwired: 1 out]
                n2660 = Build Array(i16 1 ("元素"), w3332, w3326, w3325, w3324, w3323, 0.0 ("元素")) -> (w3336:dbl[])
                n2661 = call "多帧发送机制(EV05).vi"("can卡类型"=w3340, "设备索引号"=w3339, "CAN端口"=w3338, "命令"=w3334, "板号"=u8 0, "命令序号"=w3322, "输入数据"=w3336) -> ()  [unwired: 1 in, 12 out]
              }
              frame True {
                w3350 = 256.0 ("y")
                w3342 = u32 2 ("命令序号")
                w3354 = u8 192 ("命令")
                n2662 = local read "动作保持时间"() -> (w3351:dbl)
                n2663 = Quotient & Remainder(x=w3351, y=w3350) -> (x-y*floor(x/y)=w3343:dbl, floor(x/y)=w3347:dbl)
                n2664 = Quotient & Remainder(x=w3347, y=w3350) -> (x-y*floor(x/y)=w3344:dbl, floor(x/y)=w3348:dbl)
                n2665 = Quotient & Remainder(x=w3348, y=w3350) -> (x-y*floor(x/y)=w3345:dbl, floor(x/y)=w3349:dbl)
                n2666 = local read "设备索引号"() -> (w3359:u16)
                n2667 = local read "CAN卡类型"() -> (w3360:u32)
                n2668 = local read "CAN端口"() -> (w3358:u16)
                n2669 = Boolean To (0,1)(Boolean=w3355) -> (0, 1=w3352:i16)
                n2670 = Quotient & Remainder(x=w3349, y=w3350) -> (x-y*floor(x/y)=w3346:dbl)  [unwired: 1 out]
                n2671 = Build Array(i16 1 ("元素"), w3352, w3346, w3345, w3344, w3343, 0.0 ("元素")) -> (w3356:dbl[])
                n2672 = call "多帧发送机制(EV05).vi"("can卡类型"=w3360, "设备索引号"=w3359, "CAN端口"=w3358, "命令"=w3354, "板号"=u8 0, "命令序号"=w3342, "输入数据"=w3356) -> ()  [unwired: 1 in, 12 out]
              }
            }
            n2673 = local write "命令序号"(w3314) -> ()
            n2674 = local write "命令"(w3319) -> ()
            n2675 = local write "控制1"(TRUE ("控制1")) -> ()
            n2676 = local write "写?"(FALSE ("写?")) -> ()
            n2677 = local write "消除"(TRUE ("消除")) -> ()
            n2678 = global write "EV05全局变量1.vi" "流控帧 2"(TRUE ("流控帧 2")) -> ()
            n2679 = global write "EV05全局变量1.vi" "流控帧"(FALSE ("流控帧")) -> ()
          }
          frame #2 {
            n2680 = flat-sequence {
              tunnel: [w3362] -> w3361
              tunnel: w3361 -> [w3369]
              frame #0 {
                n2681 = while {
                  tunnel: [w3363] -> w3362
                  i -> [w3367]
                  stop <- w3364 stop-if-true
                  n2682 = local read "继电器超时处理"() -> (w3363:bool)
                  n2683 = Greater Or Equal?(x=w3367, y=20) -> (x >= y?=w3365:bool)
                  n2684 = Wait Until Next ms Multiple(millisecond multiple=u32 100 ("毫秒倍数")) -> ()  [unwired: 1 out]
                  n2685 = Or(x=w3363, y=w3365) -> (x .or. y?=w3364:bool)
                }
              }
              frame #1 {
                n2686 = case shown="假" w3369 {
                  frame False {
                    n2687 = local read "DO1"() -> (w3371:bool)
                    n2688 = Not(x=w3371) -> (.not. x?=w3370:bool)
                    n2689 = local write "DO1"(w3370) -> ()
                    n2690 = One Button Dialog(message="DO控制处理超时" ("消息"), button name ("OK")="是" ("按钮名称（“确定”）")) -> ()  [unwired: 1 out]
                  }
                  frame True {
                  }
                }
              }
            }
          }
        }
      }
      event "DO2": Value Change {
        n2691 = event-data() -> ("NewVal"=w3374:bool)  [unwired: 6 out]
        n2692 = stacked-sequence {
          tunnel: w3374 -> [_ w3387 _]
          frame #0 {
            w3377 = FALSE ("清BUFF")
            n2693 = local write "继电器超时处理"(FALSE ("继电器超时处理")) -> ()
            n2694 = local write "主从选择"(enum32{"主板", "从板"}."主板" ("主从选择")) -> ()
            n2695 = local write "清BUFF"(w3377) -> ()
            n2696 = local write "正级继电器 10"(w3377) -> ()
          }
          frame #1 {
            n2697 = case shown="真" w3387 {
              selector: w3387 -> [w3402 w3422]
              tunnel: [w3401 w3421] -> w3386
              tunnel: [w3389 w3409] -> w3381
              frame False {
                w3397 = 256.0 ("y")
                w3389 = u32 2 ("命令序号")
                w3401 = u8 192 ("命令")
                n2698 = local read "动作保持时间"() -> (w3398:dbl)
                n2699 = Quotient & Remainder(x=w3398, y=w3397) -> (x-y*floor(x/y)=w3390:dbl, floor(x/y)=w3394:dbl)
                n2700 = Quotient & Remainder(x=w3394, y=w3397) -> (x-y*floor(x/y)=w3391:dbl, floor(x/y)=w3395:dbl)
                n2701 = Quotient & Remainder(x=w3395, y=w3397) -> (x-y*floor(x/y)=w3392:dbl, floor(x/y)=w3396:dbl)
                n2702 = local read "设备索引号"() -> (w3406:u16)
                n2703 = local read "CAN卡类型"() -> (w3407:u32)
                n2704 = local read "CAN端口"() -> (w3405:u16)
                n2705 = Boolean To (0,1)(Boolean=w3402) -> (0, 1=w3399:i16)
                n2706 = Quotient & Remainder(x=w3396, y=w3397) -> (x-y*floor(x/y)=w3393:dbl)  [unwired: 1 out]
                n2707 = Build Array(i16 2 ("元素"), w3399, w3393, w3392, w3391, w3390, 0.0 ("元素")) -> (w3403:dbl[])
                n2708 = call "多帧发送机制(EV05).vi"("can卡类型"=w3407, "设备索引号"=w3406, "CAN端口"=w3405, "命令"=w3401, "板号"=u8 0, "命令序号"=w3389, "输入数据"=w3403) -> ()  [unwired: 1 in, 12 out]
              }
              frame True {
                w3417 = 256.0 ("y")
                w3409 = u32 2 ("命令序号")
                w3421 = u8 192 ("命令")
                n2709 = local read "动作保持时间"() -> (w3418:dbl)
                n2710 = Quotient & Remainder(x=w3418, y=w3417) -> (x-y*floor(x/y)=w3410:dbl, floor(x/y)=w3414:dbl)
                n2711 = Quotient & Remainder(x=w3414, y=w3417) -> (x-y*floor(x/y)=w3411:dbl, floor(x/y)=w3415:dbl)
                n2712 = Quotient & Remainder(x=w3415, y=w3417) -> (x-y*floor(x/y)=w3412:dbl, floor(x/y)=w3416:dbl)
                n2713 = local read "设备索引号"() -> (w3426:u16)
                n2714 = local read "CAN卡类型"() -> (w3427:u32)
                n2715 = local read "CAN端口"() -> (w3425:u16)
                n2716 = Boolean To (0,1)(Boolean=w3422) -> (0, 1=w3419:i16)
                n2717 = Quotient & Remainder(x=w3416, y=w3417) -> (x-y*floor(x/y)=w3413:dbl)  [unwired: 1 out]
                n2718 = Build Array(i16 2 ("元素"), w3419, w3413, w3412, w3411, w3410, 0.0 ("元素")) -> (w3423:dbl[])
                n2719 = call "多帧发送机制(EV05).vi"("can卡类型"=w3427, "设备索引号"=w3426, "CAN端口"=w3425, "命令"=w3421, "板号"=u8 0, "命令序号"=w3409, "输入数据"=w3423) -> ()  [unwired: 1 in, 12 out]
              }
            }
            n2720 = local write "命令序号"(w3381) -> ()
            n2721 = local write "命令"(w3386) -> ()
            n2722 = local write "控制1"(TRUE ("控制1")) -> ()
            n2723 = local write "写?"(FALSE ("写?")) -> ()
            n2724 = local write "消除"(TRUE ("消除")) -> ()
            n2725 = global write "EV05全局变量1.vi" "流控帧 2"(TRUE ("流控帧 2")) -> ()
            n2726 = global write "EV05全局变量1.vi" "流控帧"(FALSE ("流控帧")) -> ()
          }
          frame #2 {
            n2727 = flat-sequence {
              tunnel: [w3429] -> w3428
              tunnel: w3428 -> [w3436]
              frame #0 {
                n2728 = while {
                  tunnel: [w3430] -> w3429
                  i -> [w3434]
                  stop <- w3431 stop-if-true
                  n2729 = local read "继电器超时处理"() -> (w3430:bool)
                  n2730 = Greater Or Equal?(x=w3434, y=20) -> (x >= y?=w3432:bool)
                  n2731 = Wait Until Next ms Multiple(millisecond multiple=u32 100 ("毫秒倍数")) -> ()  [unwired: 1 out]
                  n2732 = Or(x=w3430, y=w3432) -> (x .or. y?=w3431:bool)
                }
              }
              frame #1 {
                n2733 = case shown="假" w3436 {
                  frame False {
                    n2734 = local read "DO2"() -> (w3438:bool)
                    n2735 = Not(x=w3438) -> (.not. x?=w3437:bool)
                    n2736 = local write "DO2"(w3437) -> ()
                    n2737 = One Button Dialog(message="DO控制处理超时" ("消息"), button name ("OK")="是" ("按钮名称（“确定”）")) -> ()  [unwired: 1 out]
                  }
                  frame True {
                  }
                }
              }
            }
          }
        }
      }
      event "DO1 2": Value Change {
        n2738 = event-data() -> ("NewVal"=w3441:bool)  [unwired: 6 out]
        n2739 = stacked-sequence {
          tunnel: w3441 -> [_ w3455 _]
          frame #0 {
            w3444 = FALSE ("继电器超时处理")
            n2740 = local write "继电器超时处理"(w3444) -> ()
            n2741 = local write "正级继电器 11"(w3444) -> ()
            n2742 = local write "主从选择"(enum32{"主板", "从板"}."从板" ("主从选择")) -> ()
          }
          frame #1 {
            n2743 = case shown="假" w3455 {
              selector: w3455 -> [w3470 w3490]
              tunnel: [w3469 w3489] -> w3454
              tunnel: [w3468 w3488] -> w3448
              tunnel: [w3457 w3477] -> w3449
              frame True {
                w3465 = 256.0 ("y")
                w3457 = u32 2 ("命令序号")
                w3469 = u8 192 ("命令")
                n2744 = local read "动作保持时间"() -> (w3466:dbl)
                n2745 = Quotient & Remainder(x=w3466, y=w3465) -> (x-y*floor(x/y)=w3458:dbl, floor(x/y)=w3462:dbl)
                n2746 = Quotient & Remainder(x=w3462, y=w3465) -> (x-y*floor(x/y)=w3459:dbl, floor(x/y)=w3463:dbl)
                n2747 = Quotient & Remainder(x=w3463, y=w3465) -> (x-y*floor(x/y)=w3460:dbl, floor(x/y)=w3464:dbl)
                n2748 = Quotient & Remainder(x=w3464, y=w3465) -> (x-y*floor(x/y)=w3461:dbl)  [unwired: 1 out]
                n2749 = Boolean To (0,1)(Boolean=w3470) -> (0, 1=w3467:i16)
                n2750 = local read "设备索引号"() -> (w3474:u16)
                n2751 = local read "CAN卡类型"() -> (w3475:u32)
                n2752 = local read "从板板号"() -> (w3468:u8)
                n2753 = local read "CAN端口"() -> (w3473:u16)
                n2754 = Build Array(i16 3 ("元素"), w3467, w3461, w3460, w3459, w3458, 0.0 ("元素")) -> (w3472:dbl[])
                n2755 = call "多帧发送机制(EV05).vi"("can卡类型"=w3475, "设备索引号"=w3474, "CAN端口"=w3473, "命令"=w3469, "板号"=w3468, "命令序号"=w3457, "输入数据"=w3472) -> ()  [unwired: 1 in, 12 out]
              }
              frame False {
                w3485 = 256.0 ("y")
                w3477 = u32 2 ("命令序号")
                w3489 = u8 192 ("命令")
                n2756 = local read "动作保持时间"() -> (w3486:dbl)
                n2757 = Quotient & Remainder(x=w3486, y=w3485) -> (x-y*floor(x/y)=w3478:dbl, floor(x/y)=w3482:dbl)
                n2758 = Quotient & Remainder(x=w3482, y=w3485) -> (x-y*floor(x/y)=w3479:dbl, floor(x/y)=w3483:dbl)
                n2759 = Quotient & Remainder(x=w3483, y=w3485) -> (x-y*floor(x/y)=w3480:dbl, floor(x/y)=w3484:dbl)
                n2760 = Quotient & Remainder(x=w3484, y=w3485) -> (x-y*floor(x/y)=w3481:dbl)  [unwired: 1 out]
                n2761 = Boolean To (0,1)(Boolean=w3490) -> (0, 1=w3487:i16)
                n2762 = local read "设备索引号"() -> (w3494:u16)
                n2763 = local read "CAN卡类型"() -> (w3495:u32)
                n2764 = local read "从板板号"() -> (w3488:u8)
                n2765 = local read "CAN端口"() -> (w3493:u16)
                n2766 = Build Array(i16 1 ("元素"), w3487, w3481, w3480, w3479, w3478, 0.0 ("元素")) -> (w3492:dbl[])
                n2767 = call "多帧发送机制(EV05).vi"("can卡类型"=w3495, "设备索引号"=w3494, "CAN端口"=w3493, "命令"=w3489, "板号"=w3488, "命令序号"=w3477, "输入数据"=w3492) -> ()  [unwired: 1 in, 12 out]
              }
            }
            n2768 = local write "从板板号"(w3448) -> ()
            n2769 = local write "命令序号"(w3449) -> ()
            n2770 = local write "命令"(w3454) -> ()
            n2771 = local write "清BUFF"(FALSE ("清BUFF")) -> ()
            n2772 = local write "写?"(FALSE ("写?")) -> ()
            n2773 = local write "控制1"(TRUE ("控制1")) -> ()
            n2774 = global write "EV05全局变量1.vi" "流控帧"(FALSE ("流控帧")) -> ()
            n2775 = global write "EV05全局变量1.vi" "流控帧 2"(TRUE ("流控帧 2")) -> ()
            n2776 = local write "消除"(TRUE ("消除")) -> ()
          }
          frame #2 {
            n2777 = flat-sequence {
              tunnel: [w3497] -> w3496
              tunnel: w3496 -> [w3504]
              frame #0 {
                n2778 = while {
                  tunnel: [w3498] -> w3497
                  i -> [w3502]
                  stop <- w3499 stop-if-true
                  n2779 = local read "继电器超时处理"() -> (w3498:bool)
                  n2780 = Greater Or Equal?(x=w3502, y=20) -> (x >= y?=w3500:bool)
                  n2781 = Wait Until Next ms Multiple(millisecond multiple=u32 100 ("毫秒倍数")) -> ()  [unwired: 1 out]
                  n2782 = Or(x=w3498, y=w3500) -> (x .or. y?=w3499:bool)
                }
              }
              frame #1 {
                n2783 = case shown="假" w3504 {
                  frame False {
                    n2784 = local read "DO1 2"() -> (w3506:bool)
                    n2785 = Not(x=w3506) -> (.not. x?=w3505:bool)
                    n2786 = local write "DO1 2"(w3505) -> ()
                    n2787 = One Button Dialog(message="DO控制处理超时" ("消息"), button name ("OK")="是" ("按钮名称（“确定”）")) -> ()  [unwired: 1 out]
                  }
                  frame True {
                  }
                }
              }
            }
          }
        }
      }
      event "读取转换为写入": Value Change {
        n2788 = event-data() -> ("NewVal"=w3509:bool)  [unwired: 6 out]
        n2789 = case shown="真" w3509 {
          tunnel: w3513 -> [w3515 w3520]
          tunnel: [w3515 w3519] -> w3512
          tunnel: w3511 -> [w3514 w3518]
          tunnel: [w3514 w3517] -> w3510
          frame False {
          }
          frame True {
            n2790 = Enqueue Element(queue=w3520, element="读取转换为写入", error in (no error)=w3518) -> (queue out=w3519:refnum<queue>, error out=w3517:errorcluster)  [unwired: 2 out]
          }
        }
      }
      event "读取故障详细状态": Value Change {
        n2791 = event-data() -> ("NewVal"=w3525:bool)  [unwired: 5 out]
        n2792 = case shown="真" w3525 {
          tunnel: w3524 -> [w3527 w3540]
          tunnel: w3523 -> [w3526 w3539]
          tunnel: [w3527 w3538] -> w3522
          tunnel: [w3526 w3537] -> w3521
          frame False {
          }
          frame True {
            n2793 = disable-structure shown="启用" {
              disable-tunnel: [w3549 TRUE ("发送成功")] -> w3536
              frame Disabled {
                n2794 = local read "主从选择"() -> (w3541:enum32{"主板", "从板"})
                n2795 = case shown="\"主板\", 默认" w3541 {
                  tunnel: [0.0 ("FUNC") w3551] -> w3546
                  frame "主板", Default {
                  }
                  frame "从板" {
                    n2796 = local read "从板号"() -> (w3551:u8)
                  }
                }
                n2797 = local read "设备索引号"() -> (w3543:u16)
                n2798 = local read "CAN卡类型"() -> (w3544:u32)
                n2799 = local read "CAN端口"() -> (w3542:u16)
                n2800 = call "标定授权发送.vi"("CAN卡类型"=w3544, "解锁类型"=enum16{"读取", "写", "下载"}."写", "设备索引号"=w3543, "CAN端口"=w3542, "是否连接"=TRUE, "板选择"=0, "FUNC"=w3546) -> ("发送成功"=w3549:bool)  [unwired: 8 out]
              }
              frame Enabled {
              }
            }
            n2801 = case shown="真" w3536 {
              tunnel: w3540 -> [w3554 w3559]
              tunnel: w3539 -> [w3553 w3558]
              tunnel: [w3554 w3556] -> w3538
              tunnel: [w3553 w3555] -> w3537
              frame False {
              }
              frame True {
                n2802 = Enqueue Element(queue=w3559, element="读取故障状态" ("元素"), error in (no error)=w3558) -> (queue out=w3556:refnum<queue>, error out=w3555:errorcluster)  [unwired: 2 out]
              }
            }
            n2803 = local write "电池故障"(string[][] []) -> ()
            n2804 = global write "EV05全局变量1.vi" "流控帧 2"(TRUE ("流控帧")) -> ()
            n2805 = local write "写?"(FALSE ("写?")) -> ()
            n2806 = local write "控制1"(TRUE ("控制1")) -> ()
            n2807 = local write "消除"(TRUE ("消除")) -> ()
            n2808 = local write "清BUFF"(FALSE ("清BUFF")) -> ()
            n2809 = global write "EV05全局变量1.vi" "流控帧"(FALSE ("流控帧")) -> ()
            n2810 = call <vilib>:"Set Busy.vi"("disable click? (T)"=FALSE) -> ()  [unwired: 3 in, 8 out]
          }
        }
      }
      event "项目软本读取": Value Change {
        n2811 = event-data() -> ("NewVal"=w3564:bool)  [unwired: 5 out]
        n2812 = case shown="真" w3564 {
          tunnel: w3563 -> [w3566 w3573]
          tunnel: w3562 -> [w3565 w3572]
          tunnel: [w3566 w3571] -> w3561
          tunnel: [w3565 w3570] -> w3560
          frame False {
          }
          frame True {
            n2813 = global read "EV05全局变量1.vi" "授权功能"() -> (w3568:bool)
            n2814 = case shown="假" w3568 {
              tunnel: [TRUE ("发送成功") w3592] -> w3569
              frame False {
              }
              frame True {
                n2815 = local read "设备索引号"() -> (w3587:u16)
                n2816 = local read "CAN卡类型"() -> (w3588:u32)
                n2817 = local read "CAN端口"() -> (w3586:u16)
                n2818 = call "标定授权发送.vi"("CAN卡类型"=w3588, "解锁类型"=enum16{"读取", "写", "下载"}."读取", "设备索引号"=w3587, "CAN端口"=w3586, "是否连接"=TRUE, "板选择"=0, "FUNC"=u32 0) -> ("发送成功"=w3592:bool)  [unwired: 8 out]
              }
            }
            n2819 = stacked-sequence {
              tunnel: [w3576] -> w3567
              frame #0 {
                w3576 = FALSE ("disable click? (T)")
                w3579 = FALSE ("写?")
                n2820 = local write "写?"(w3579) -> ()
                n2821 = global write "EV05全局变量1.vi" "写入超时"(w3579) -> ()
                n2822 = local write "项目软件版本号"(" " ("项目软件版本号")) -> ()
                n2823 = global write "EV05全局变量1.vi" "流控帧"(FALSE ("流控帧")) -> ()
                n2824 = local write "主从选择"(enum32{"主板", "从板"}."主板" ("主从选择")) -> ()
                n2825 = call <vilib>:"Set Busy.vi"("disable click? (T)"=w3576) -> ()  [unwired: 3 in, 8 out]
                n2826 = local write "清BUFF"(FALSE ("清BUFF")) -> ()
                n2827 = property on="保存版本信息" class="Bool (严格)"("Visible"=TRUE ("可见")) -> ()  [unwired: 2 in, 2 out]
                n2828 = global write "EV05全局变量1.vi" "流控帧 2"(TRUE ("流控帧 2")) -> ()
                n2829 = local write "控制1"(TRUE ("控制1")) -> ()
                n2830 = local write "消除"(TRUE ("消除")) -> ()
              }
            }
            n2831 = case shown="真" w3569 {
              tunnel: w3573 -> [w3594 w3599]
              tunnel: w3572 -> [w3593 w3598]
              tunnel: [w3594 w3596] -> w3571
              tunnel: [w3593 w3595] -> w3570
              tunnel: w3567 -> [_ _]
              frame False {
              }
              frame True {
                n2832 = Enqueue Element(queue=w3599, element="项目软件版本读取" ("元素"), error in (no error)=w3598) -> (queue out=w3596:refnum<queue>, error out=w3595:errorcluster)  [unwired: 2 out]
              }
            }
          }
        }
      }
      event "读硬件版本号": Value Change {
        n2833 = event-data() -> ("NewVal"=w3604:bool)  [unwired: 5 out]
        n2834 = case shown="真" w3604 {
          tunnel: w3603 -> [w3606 w3613]
          tunnel: w3602 -> [w3605 w3612]
          tunnel: [w3606 w3611] -> w3601
          tunnel: [w3605 w3610] -> w3600
          frame False {
          }
          frame True {
            n2835 = global read "EV05全局变量1.vi" "授权功能"() -> (w3608:bool)
            n2836 = case shown="假" w3608 {
              tunnel: [TRUE ("发送成功") w3632] -> w3609
              frame False {
              }
              frame True {
                n2837 = local read "设备索引号"() -> (w3627:u16)
                n2838 = local read "CAN卡类型"() -> (w3628:u32)
                n2839 = local read "CAN端口"() -> (w3626:u16)
                n2840 = call "标定授权发送.vi"("CAN卡类型"=w3628, "解锁类型"=enum16{"读取", "写", "下载"}."读取", "设备索引号"=w3627, "CAN端口"=w3626, "是否连接"=TRUE, "板选择"=0, "FUNC"=u32 0) -> ("发送成功"=w3632:bool)  [unwired: 8 out]
              }
            }
            n2841 = stacked-sequence {
              tunnel: [w3616] -> w3607
              frame #0 {
                w3616 = TRUE ("控制1")
                w3620 = FALSE ("写?")
                n2842 = local write "写?"(w3620) -> ()
                n2843 = global write "EV05全局变量1.vi" "写入超时"(w3620) -> ()
                n2844 = call <vilib>:"Set Busy.vi"("disable click? (T)"=FALSE) -> ()  [unwired: 3 in, 8 out]
                n2845 = local write "硬件版本号"("" ("硬件版本号")) -> ()
                n2846 = property on="保存版本信息" class="Bool (严格)"("Visible"=TRUE ("可见")) -> ()  [unwired: 2 in, 2 out]
                n2847 = local write "主从选择"(enum32{"主板", "从板"}."主板" ("主从选择")) -> ()
                n2848 = local write "控制1"(w3616) -> ()
                n2849 = local write "清BUFF"(FALSE ("清BUFF")) -> ()
                n2850 = global write "EV05全局变量1.vi" "流控帧 2"(TRUE ("流控帧 2")) -> ()
                n2851 = local write "消除"(TRUE ("消除")) -> ()
                n2852 = global write "EV05全局变量1.vi" "流控帧"(FALSE ("流控帧")) -> ()
              }
            }
            n2853 = case shown="真" w3609 {
              tunnel: w3613 -> [w3634 w3639]
              tunnel: w3612 -> [w3633 w3638]
              tunnel: [w3634 w3636] -> w3611
              tunnel: [w3633 w3635] -> w3610
              tunnel: w3607 -> [_ _]
              frame False {
              }
              frame True {
                n2854 = Enqueue Element(queue=w3639, element="硬件版本读取" ("元素"), error in (no error)=w3638) -> (queue out=w3636:refnum<queue>, error out=w3635:errorcluster)  [unwired: 2 out]
              }
            }
          }
        }
      }
      event "平台软件版本读取": Value Change {
        n2855 = event-data() -> ("NewVal"=w3644:bool)  [unwired: 5 out]
        n2856 = case shown="真" w3644 {
          tunnel: w3643 -> [w3646 w3653]
